vi "PtByPt and Array Based Filter.vi"() -> ()   [LabVIEW 2023]
doc: "Compares Point By Point filters with array-based filters. The Point By Point filter works in real-time and online while the array-based filter waits for the array to be compiled first. Array-based filter is also called block filter."
uses:
  <vilib>/Analysis/3filter.llb/Butterworth Filter (DBL).vi
  <vilib>/ptbypt/NI_PtbyPt.lvlib
  <vilib>/Analysis/NI_AALBase.lvlib
panel:
  in  "noise level":dbl(slide)=0.2 scale=0.0..5.0
  in  "Initialize Array-based filter":bool
  out "Signal (sine plus noise)":dbl(graph)=1.8684475367496631
  out "Filtered Signal (Array Based)":dbl[](graph)
  in  "Stop":bool
  out "Filtered Signal (Point-By-Point)":dbl(graph)=2.18622070078109
  # "Overview: Compares Point By Point filters with array-based filters.\nRequirement: LabVIEW Full Development System\nInstructions:\n1. Run the VI.\n2. Change the noise level and observe the results in the Filtered Signal graphs.\n3. Click Stop to stop the VI."
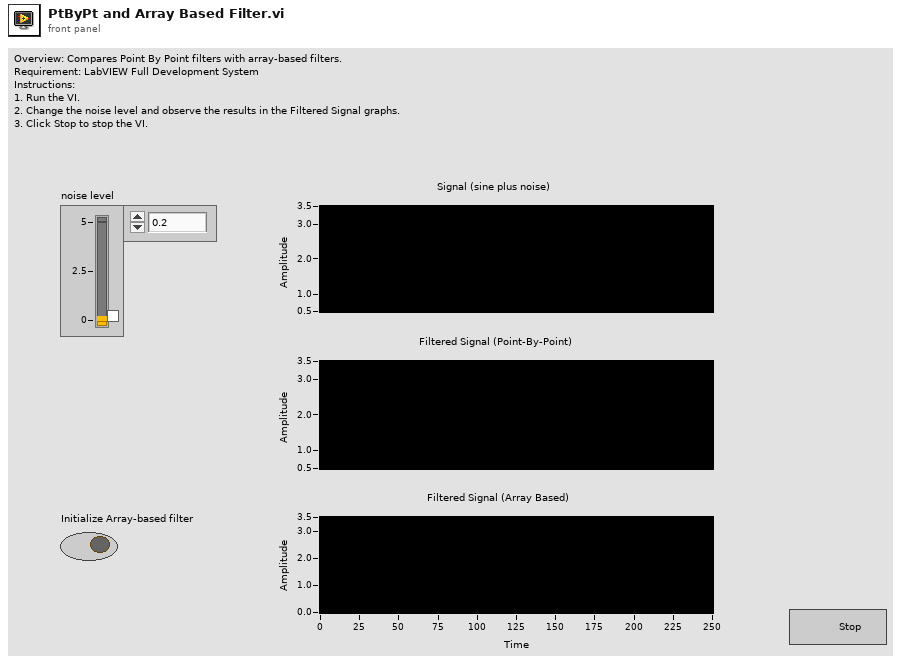
[diagram p1: front panel]
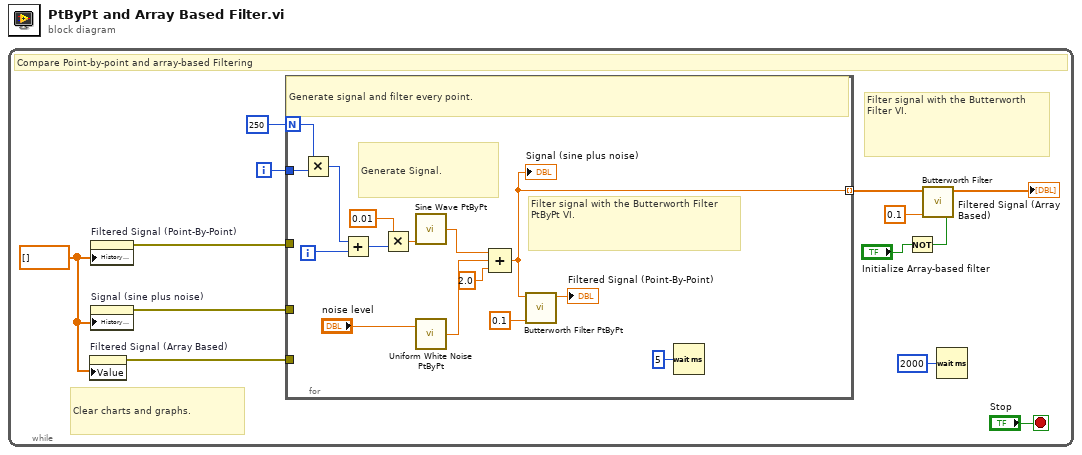
[diagram p0: block diagram]
diagram:
  n1 = while {
    i -> [w11]
    stop <- "Stop" stop-if-true
    w1 = dbl[] [] ("Output Array")
    # "Clear charts and graphs."
    # "Filter signal with the Butterworth Filter VI."
    # "Compare Point-by-point and array-based Filtering"
    n2 = property on="Filtered Signal (Array Based)" class="WFGraph (strict)"("Value"=w1) -> (error out=w7:errorcluster)  [unwired: 2 in, 1 out]
    n3 = property on="Filtered Signal (Point-By-Point)" class="WFChart (strict)"("History Data"=w1) -> (error out=w9:errorcluster)  [unwired: 2 in, 1 out]
    n4 = property on="Signal (sine plus noise)" class="WFChart (strict)"("History Data"=w1) -> (error out=w8:errorcluster)  [unwired: 2 in, 1 out]
    n5 = for {
      N: 250 -> [w24]
      tunnel: [w21] -> w12 mode=indexing
      tunnel: w11 -> [w23]
      tunnel: w9 -> [_]
      tunnel: w8 -> [_]
      tunnel: w7 -> [_]
      i -> [w28]
      # "Generate Signal."
      # "Filter signal with the Butterworth Filter PtByPt VI."
      # "Generate signal and filter every point."
      n6 = Multiply(x=w24, y=w23) -> (x*y=w22:i32)
      n7 = Add(x=w22, y=w28) -> (x+y=w18:i32)
      n8 = Multiply(x=0.01, y=w18) -> (x*y=w27:dbl)
      n9 = call <vilib>:"Sine Wave PtByPt.vi"("time"=w27) -> ("sine wave"=w16:dbl)  [unwired: 3 in]
      n10 = call <vilib>:"Uniform White Noise PtByPt.vi"("amplitude"="noise level") -> ("uniform white noise"=w15:dbl)  [unwired: 2 in]
      n11 = Compound Arithmetic op=ADD(w16, w15, 2.0) -> (w21:dbl)
      "Signal (sine plus noise)" <- w21
      n12 = call <vilib>:"Butterworth Filter PtByPt.vi"("low cutoff freq: fl"=0.1, "x"=w21) -> ("Filtered x"=→"Filtered Signal (Point-By-Point)":dbl)  [unwired: 7 in, 1 out]
      n13 = Wait (ms)(milliseconds to wait=u32 5) -> ()  [unwired: 1 out]
    }
    n14 = Not(x="Initialize Array-based filter") -> (.not. x?=w5:bool)
    n15 = call-poly <vilib>:"Butterworth Filter.vi"("init/cont (init:F)"=w5, "low cutoff freq: fl"=0.1, "X"=w12) -> ("Filtered X"=→"Filtered Signal (Array Based)":dbl[])  [unwired: 5 in, 1 out]
    n16 = Wait (ms)(milliseconds to wait=u32 2000) -> ()  [unwired: 1 out]
  }
